vi "Timed Write to Hardware.vi"(7 "Valid triggers":bool, 8 "error in":errorcluster, 9 "Trigger Values":dbl[](array[numeric]), 10 "Values":dbl[](array[numeric]), 11 "Execution Unit in":refnum<class "Execution Unit.lvclass">) -> (0 "error out":errorcluster, 1 "Trigger Values out":dbl[](array[numeric]), 2 "Values out":dbl[](array[numeric]), 3 "Execution Unit out":refnum<class "Execution Unit.lvclass">)   [LabVIEW 2020, in "Ballard ARINC 429 Engine.lvlib" / "Custom Device.lvlib"]
uses:
  Custom Device.lvlib
  Interfaces/Execution Unit/Execution Unit.lvclass
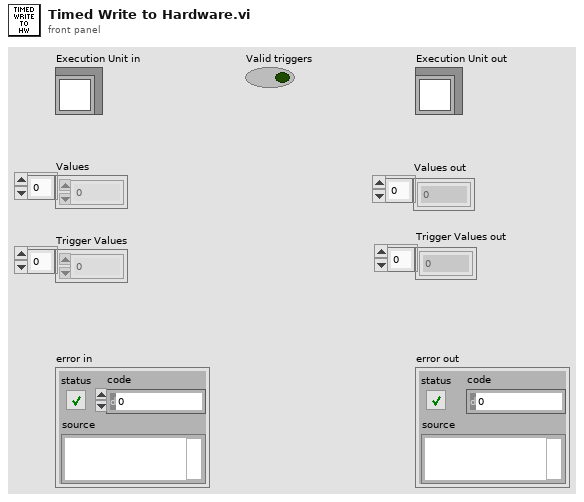
[diagram p1: front panel]
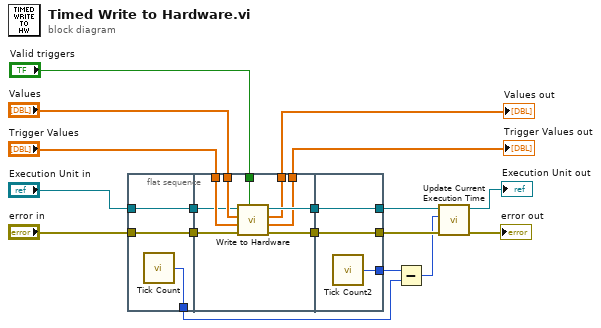
[diagram p0: block diagram]
diagram:
  n1 = flat-sequence {
    tunnel: "Execution Unit in" -> [w20]
    tunnel: "error in" -> [w21]
    tunnel: [w21] -> w10
    tunnel: [w20] -> w9
    tunnel: [w19] -> w2
    tunnel: "Valid triggers" -> [w30]
    tunnel: "Trigger Values" -> [w28]
    tunnel: "Values" -> [w26]
    tunnel: [w23] -> w12
    tunnel: [w22] -> w11
    tunnel: w10 -> [w27]
    tunnel: w9 -> [w24]
    tunnel: [w29] -> w8
    tunnel: [w25] -> w7
    tunnel: [w32] -> w14
    tunnel: [w33] -> w5
    tunnel: w8 -> [w33]
    tunnel: w7 -> [w32]
    tunnel: [w31] -> w3
    frame #0 {
      n2 = call "Tick Count"() -> ("Tick Count(uSec)"=w19:u32)
    }
    frame #1 {
      n3 = call-dynamic "Write to Hardware.vi"("valid triggers"=w30, "error in"=w27, "trigger values"=w28, "values in"=w26, "execution unit in"=w24) -> ("error out"=w29:errorcluster, "trigger values out"=w22:dbl[], "values out"=w23:dbl[], "execution unit out"=w25:refnum<class "Execution Unit.lvclass">)  [unwired: 3 in]
    }
    frame #2 {
      n4 = call "Tick Count2"() -> ("Tick Count(uSec)"=w31:u32)
    }
  }
  n5 = Subtract(x=w3, y=w2) -> (x-y=w1:u32)
  n6 = call-dynamic "Update Current Execution Time.vi"("error in"=w5, "Current Execution Time (us)"=w1, "Execution Unit in"=w14) -> ("error out"=→"error out":errorcluster, "Execution Unit out"=→"Execution Unit out":refnum<class "Execution Unit.lvclass">)  [unwired: 7 in]
  "Values out" <- w12
  "Trigger Values out" <- w11
